vi "Advance past whitespace.vi"(4 "Past Colon":bool, 6 "Past Comma":bool, 7 "JSON":string, 9 "Offset":i32, 11 "Parser State in":T1=enum."Leading Whitespace") -> (0 "Comma Not Found":bool, 1 "Offset of first non-whitespace":i32, 3 "Parser State":T1)   [LabVIEW 2024, in "JSONtext.lvlib"]
uses:
  JSONtext.lvlib
  Parsing State.ctl
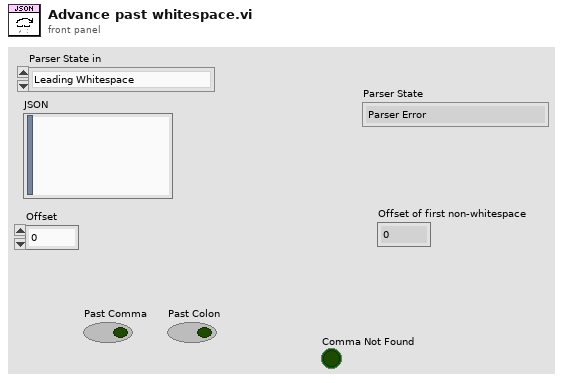
[diagram p1: front panel]
types:
  T1 = typedef "JSONtext.lvlib/Parsing State.ctl" = enum16{"Parser Error", "Object", "Array", "String", "Number/Other", "Leading Whitespace", "Object end", "Array end", "Value end"}
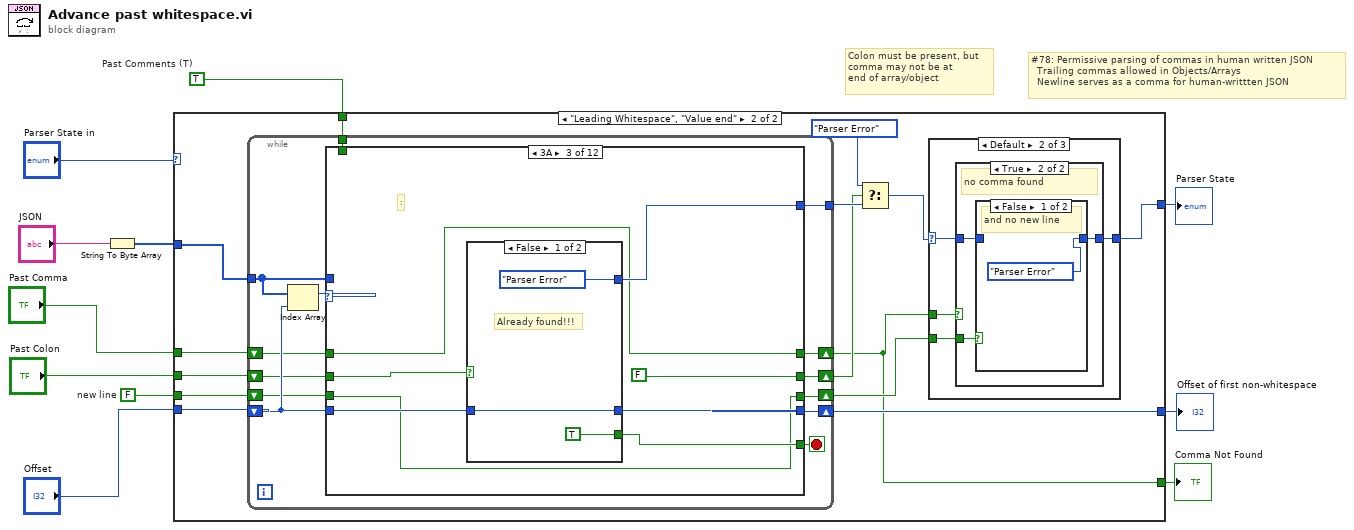
[diagram p0: block diagram]
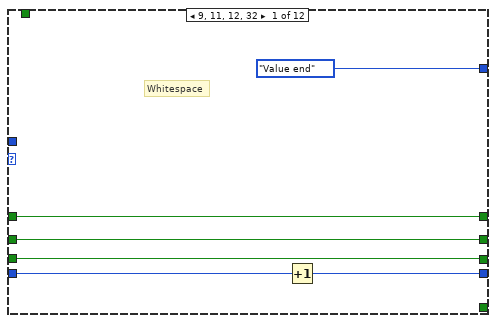
[diagram p7: hidden frame]
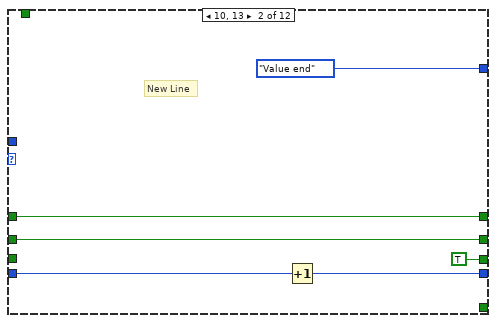
[diagram p8: hidden frame]
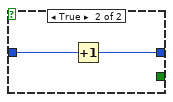
[diagram p9: hidden frame]
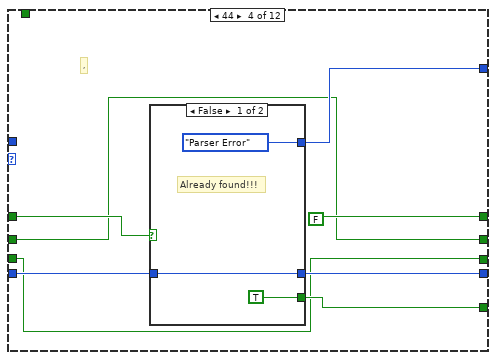
[diagram p10: hidden frame]
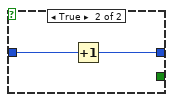
[diagram p11: hidden frame]
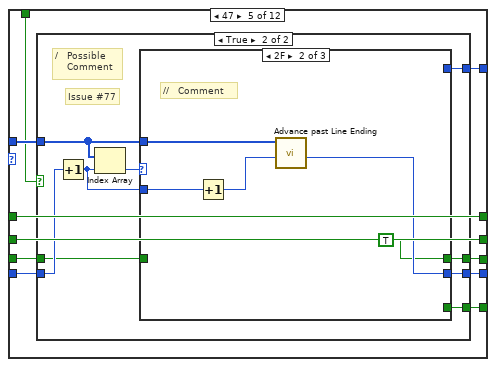
[diagram p12: hidden frame]
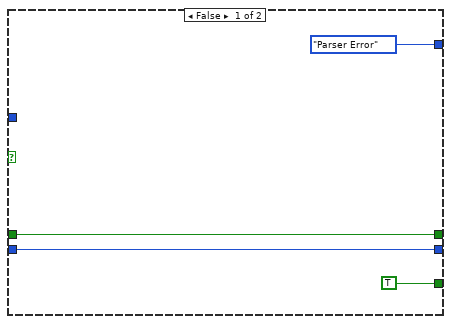
[diagram p13: hidden frame]
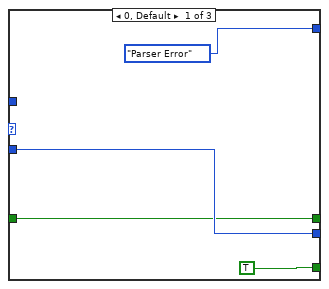
[diagram p14: hidden frame]
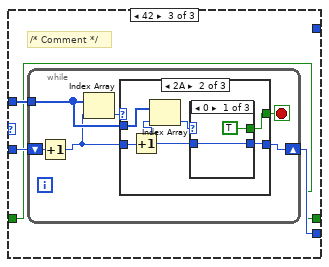
[diagram p15: hidden frame]
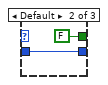
[diagram p17: hidden frame]
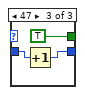
[diagram p18: hidden frame]
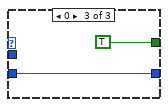
[diagram p19: hidden frame]
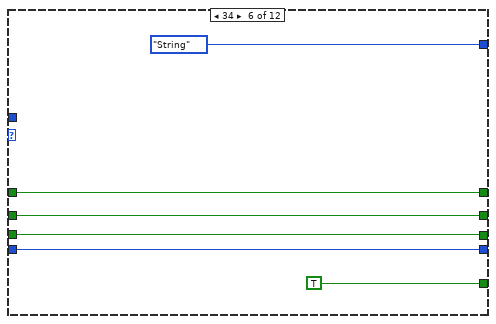
[diagram p20: hidden frame]
diagram:
  w2 = FALSE  # new line
  w3 = TRUE  # Past Comments (T)
  # "#78: Permissive parsing of commas in human written JSON\n  Trailing commas allowed in Objects/Arrays\n  Newline serves as a comma for human-writtten JSON"
  # "Colon must be present, but\ncomma may not be at\nend of array/object"
  n1 = String To Byte Array(string="JSON") -> (unsigned byte array=w5:u8[])
  n2 = case shown="\"Leading Whitespace\", \"Value end\"" "Parser State in" {
    selector: "Parser State in" -> [w13 _]
    tunnel: [w13 w27] -> w11
    tunnel: [w12 w26] -> w10
    tunnel: "Offset" -> [w12 w25]
    tunnel: w5 -> [_ w18]
    tunnel: "Past Comma" -> [_ w24]
    tunnel: "Past Colon" -> [_ w23]
    tunnel: w3 -> [_ w17]
    tunnel: w2 -> [_ w16]
    tunnel: [_ w14] -> w1
    frame "Parser Error", Default {
    }
    frame "Leading Whitespace", "Value end" {
      n3 = while {
        tunnel: w18 -> [w43]
        shift-right: [w48] -> w26
        shift-left: w25 -> [w49]
        tunnel: [w51] -> w22
        shift-right: [w47] -> w14
        shift-left: w24 -> [w46]
        shift-right: [w44] -> w20
        shift-left: w23 -> [w45]
        tunnel: w17 -> [w42]
        shift-right: [w40] -> w15
        shift-left: w16 -> [w41]
        stop <- w50 stop-if-true
        n4 = Index Array(array=w43, index=w49) -> (element=w52:u8)
        n5 = case shown="3A" w52 {
          tunnel: [Parsing_State."Value end" Parsing_State."Value end" w70 w83 w95 Parsing_State."String" Parsing_State."Number/Other" Parsing_State."Array" Parsing_State."Array end" Parsing_State."Object" Parsing_State."Object end" Parsing_State."Parser Error"] -> w51
          tunnel: [_ _ w69 w82 w94 TRUE TRUE TRUE TRUE TRUE TRUE TRUE] -> w50
          tunnel: w49 -> [w58 w64 w72 w85 w98 w152 w158 w164 w170 w176 w182 w190]
          tunnel: [w57 w63 w71 w84 w96 w152 w158 w164 w170 w176 w182 w190] -> w48
          tunnel: [w55 w61 w66 FALSE ("Allow Comma") w100 w151 w157 w163 w169 w175 w181 w187] -> w47
          tunnel: w46 -> [w55 w61 w66 w81 w100 w151 w157 w163 w169 w175 w181 w187]
          tunnel: [w54 w60 FALSE ("Allow Comma") w79 w99 w150 w156 w162 w168 w174 w180 w186] -> w44
          tunnel: w45 -> [w54 w60 w68 w79 w99 w150 w156 w162 w168 w174 w180 w186]
          tunnel: w43 -> [_ _ _ _ w97 _ _ _ _ _ _ _]
          tunnel: w42 -> [_ _ _ _ w93 _ _ _ _ _ _ _]
          tunnel: w41 -> [w53 _ w65 w78 w92 w149 w155 w161 w167 w173 w179 w185]
          tunnel: [w53 TRUE w65 w78 w91 w149 w155 w161 w167 w173 w179 w185] -> w40
          frame 9, 11, 12, 32 {
            # "Whitespace"
            n6 = Increment(x=w58) -> (x+1=w57:i32)
          }
          frame 10, 13 {
            # "New Line"
            n7 = Increment(x=w64) -> (x+1=w63:i32)
          }
          frame 58 {
            # ":"
            n8 = case shown="False" w68 {
              tunnel: w72 -> [w74 w77]
              tunnel: [w74 w76] -> w71
              tunnel: [Parsing_State."Parser Error" _] -> w70
              tunnel: [TRUE _] -> w69
              frame False {
                # "Already found!!!"
              }
              frame True {
                n9 = Increment(x=w77) -> (x+1=w76:i32)
              }
            }
          }
          frame 44 {
            # ","
            n10 = case shown="False" w81 {
              tunnel: w85 -> [w87 w90]
              tunnel: [w87 w89] -> w84
              tunnel: [Parsing_State."Parser Error" _] -> w83
              tunnel: [TRUE _] -> w82
              frame False {
                # "Already found!!!"
              }
              frame True {
                n11 = Increment(x=w90) -> (x+1=w89:i32)
              }
            }
          }
          frame 47 {
            n12 = case shown="True" w93 {
              tunnel: w98 -> [w103 w113]
              tunnel: w97 -> [_ w111]
              tunnel: [w103 w109] -> w96
              tunnel: [Parsing_State."Parser Error" ("t") w108] -> w95
              tunnel: [TRUE w107] -> w94
              tunnel: w92 -> [w101 w106]
              tunnel: [w101 w105] -> w91
              frame False {
              }
              frame True {
                # "Issue #77"
                # "/   Possible \n    Comment"
                n13 = Increment(x=w113) -> (x+1=w110:i32)
                n14 = Index Array(array=w111, index=w110) -> (element=w112:u8)
                n15 = case shown="2F" w112 {
                  tunnel: w111 -> [_ w122 w126]
                  tunnel: w110 -> [w115 w121 w124]
                  tunnel: [w115 w120 w125] -> w109
                  tunnel: [Parsing_State."Parser Error" ("t") _ _] -> w108
                  tunnel: [TRUE _ _] -> w107
                  tunnel: w106 -> [w114 _ w123]
                  tunnel: [w114 TRUE w123] -> w105
                  frame 0, Default {
                  }
                  frame 47 {
                    # "//   Comment"
                    n16 = Increment(x=w121) -> (x+1=w119:i32)
                    n17 = call "Advance past Line Ending.vi"("Offset"=w119, "JSON"=w122) -> ("Offset after Line Ending"=w120:i32)  [unwired: 9 in]
                  }
                  frame 42 {
                    # "/* Comment */"
                    n18 = while {
                      tunnel: w126 -> [w129]
                      shift-right: [w130] -> w125
                      shift-left: w124 -> [w128]
                      stop <- w131 stop-if-true
                      n19 = Increment(x=w128) -> (x+1=w127:i32)
                      n20 = Index Array(array=w129, index=w127) -> (element=w132:u8)
                      n21 = case shown="2A" w132 {
                        tunnel: w127 -> [w133 w137 w148]
                        tunnel: [_ w134 TRUE] -> w131
                        tunnel: [w133 w135 w148] -> w130
                        tunnel: w129 -> [_ w136 _]
                        frame Default {
                        }
                        frame 42 {
                          n22 = Increment(x=w137) -> (x+1=w138:i32)
                          n23 = Index Array(array=w136, index=w138) -> (element=w139:u8)
                          n24 = case shown="0" w139 {
                            tunnel: [TRUE FALSE TRUE] -> w134
                            tunnel: w138 -> [w141 w143 w145]
                            tunnel: [w141 w143 w144] -> w135
                            frame 0 {
                            }
                            frame Default {
                            }
                            frame 47 {
                              n25 = Increment(x=w145) -> (x+1=w144:i32)
                            }
                          }
                        }
                        frame 0 {
                        }
                      }
                    }
                  }
                }
              }
            }
          }
          frame 34 {
          }
          frame 43, 45, 46, 48..57, 69, 73, 78, 101, 102, 110, 116 {
          }
          frame 91 {
          }
          frame 93 {
          }
          frame 123 {
          }
          frame 125 {
          }
          frame Default {
          }
        }
      }
      n26 = Select(t=Parsing_State."Parser Error", s=w20, f=w22) -> (s? t:f=w19:T1)
      n27 = case shown="Default" w19 {
        selector: w19 -> [w28 w30 w39]
        tunnel: [w28 w31 w39] -> w27
        tunnel: w14 -> [_ w32 _]
        tunnel: w15 -> [_ w29 _]
        frame "Parser Error" {
        }
        frame Default {
          n28 = case shown="True" w32 {
            tunnel: [w33 w34] -> w31
            tunnel: w30 -> [w33 w35]
            tunnel: w29 -> [_ w36]
            frame False {
            }
            frame True {
              # "no comma found"
              n29 = case shown="False" w36 {
                tunnel: w35 -> [_ w38]
                tunnel: [Parsing_State."Parser Error" ("t") w38] -> w34
                frame False {
                  # "and no new line"
                }
                frame True {
                  # "Counts as a\ncomma"
                  # "but new line"
                }
              }
            }
          }
        }
        frame "Object end", "Array end" {
          # "At Object or Array end\nwe usually have no comma\nbut accept a comma"
        }
      }
    }
  }
  "Parser State" <- w11
  "Offset of first non-whitespace" <- w10
  "Comma Not Found" <- w1
